vi "GenINI_Main.vi"() -> ()   [LabVIEW 2009]
uses:
  Typedefs/GenINI_Key_Values.ctl
  Typedefs/GenINI_Read_Types.ctl
  Queue/Queue_Type.ctl
  <vilib>/Utility/miscctls.llb/LVPointTypeDef.ctl
panel:
  in  "Exit":bool
  in  "Main Tab":enum32{"Main", "Debug"}(tab)
  in  "Guess types?":bool
  in  "Generate_Typedef":bool
  in  "Generate_Code":bool
  in  "INI file":path=path "C:/"
  in  "Read_INI":bool
  in  "INI read results":T1[](array[typedef])
  in  "error in (no error)":errorcluster
  out "error out":errorcluster
  # "Version: 0.1.0"
  # "1. Select the existing INI file"
  # "2. Set the type for each key, then..."
  # "Name: GenINI\nAuthor: Joe Zoller\nLatest update: Feb. 13th, 2010\nCategory: Scripting\nVersion: 0.1.0\nLabVIEW Version: 2009\nLicense Type: BSD"
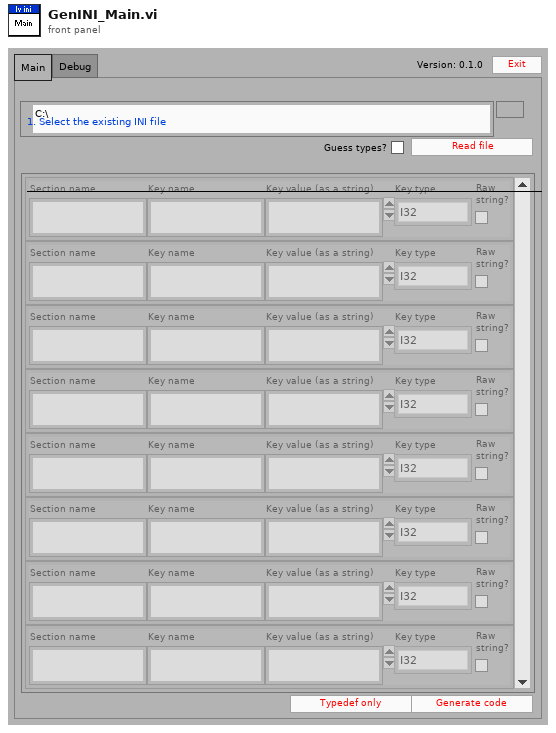
[diagram p1: front panel]
types:
  T1 = typedef "GenINI_Key_Values.ctl" = cluster{"Section name":string, "Key name":string, "Key value (as a string)":string, "Key type":T2, "Raw\nstring?":bool}
  T2 = typedef "GenINI_Read_Types.ctl" = enum16{"Boolean", "Double", "I32", "Path", "String", "U32"}
  T3 = cluster{"typedef path":path, "INI read results":T1[]}
  T4 = typedef "Queue_Type.ctl" = cluster{"cmd":string, "data":variant}
  T5 = typedef "LVPointTypeDef.ctl" = cluster{"Horizontal":i16, "Vertical":i16}
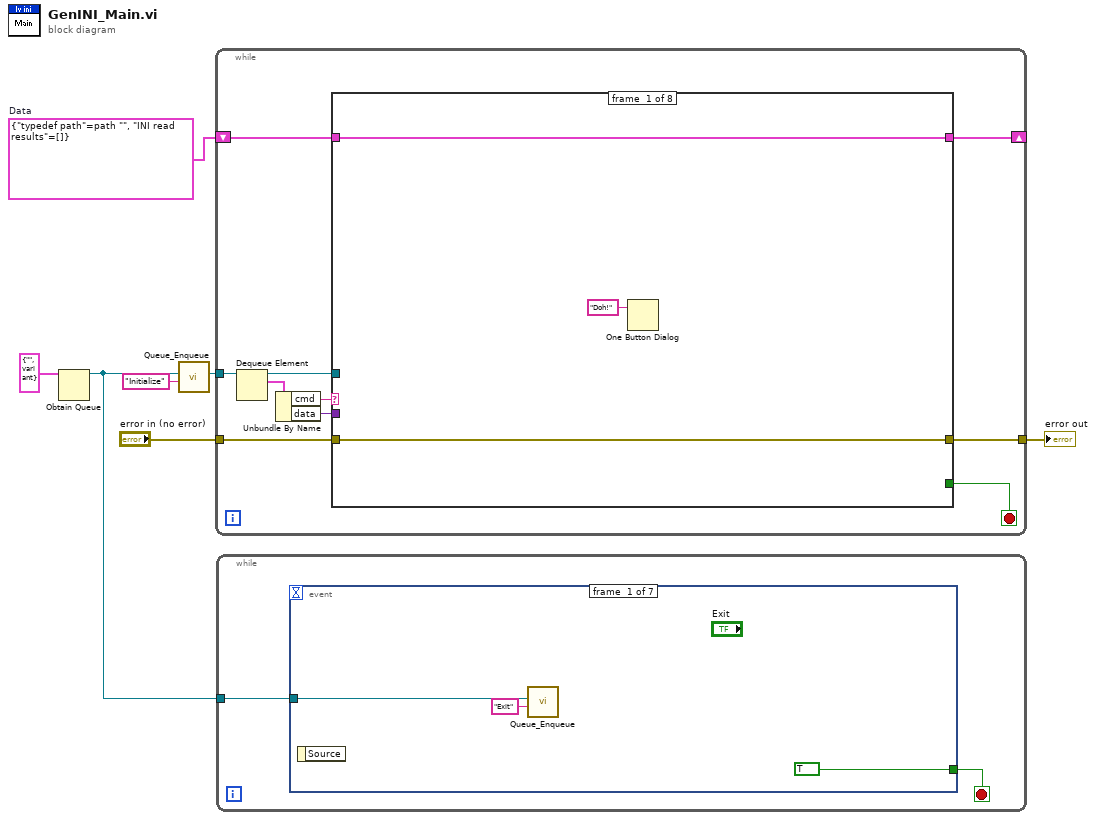
[diagram p0: block diagram]
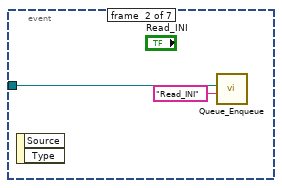
[diagram p2: hidden frame]
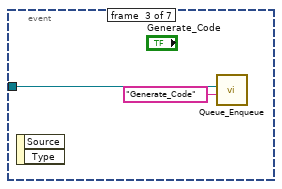
[diagram p3: hidden frame]
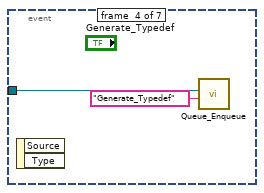
[diagram p4: hidden frame]
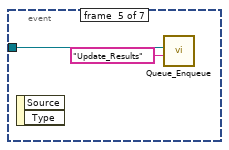
[diagram p5: hidden frame]
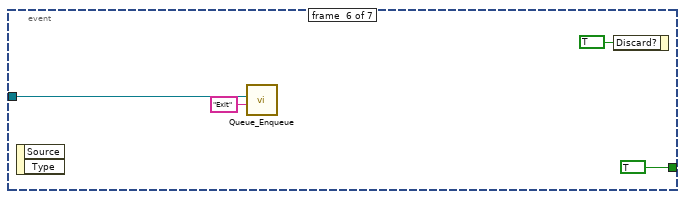
[diagram p6: hidden frame]
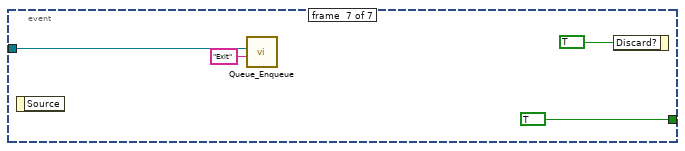
[diagram p7: hidden frame]
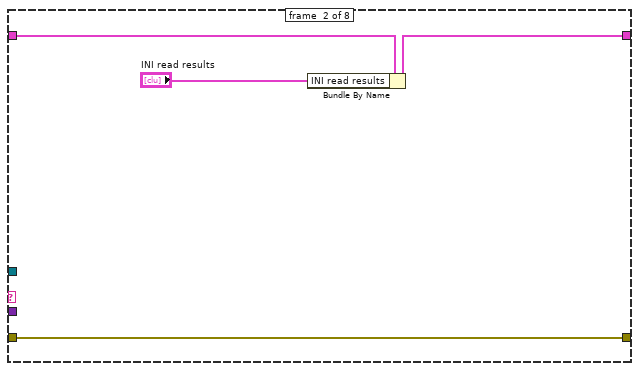
[diagram p8: hidden frame]
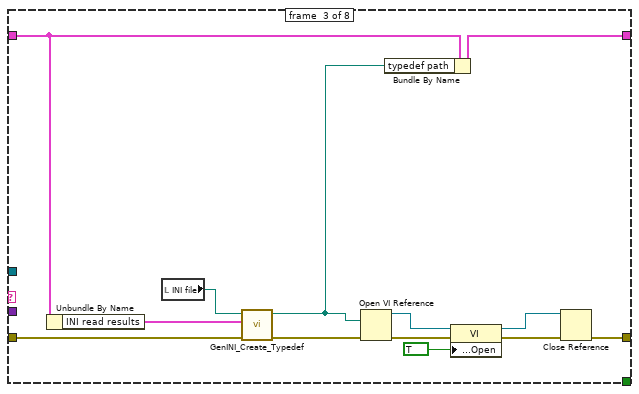
[diagram p9: hidden frame]
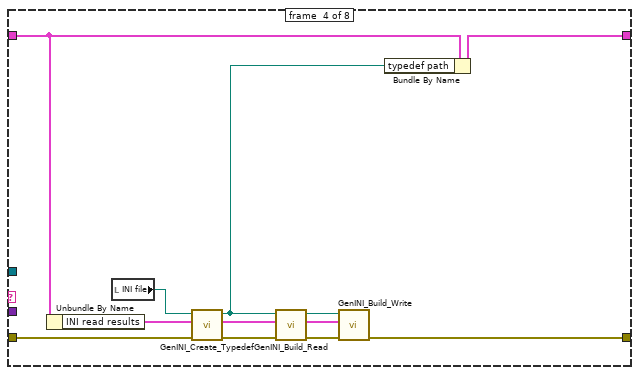
[diagram p10: hidden frame]
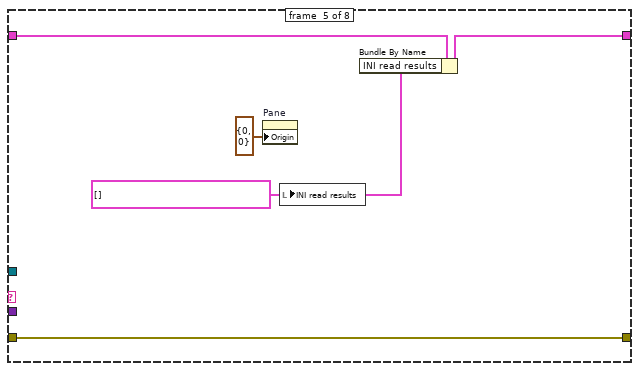
[diagram p11: hidden frame]
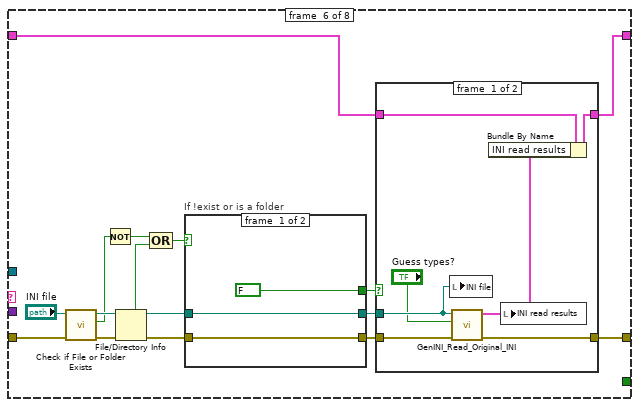
[diagram p12: hidden frame]
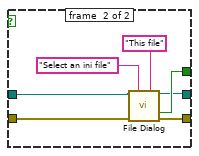
[diagram p13: hidden frame]
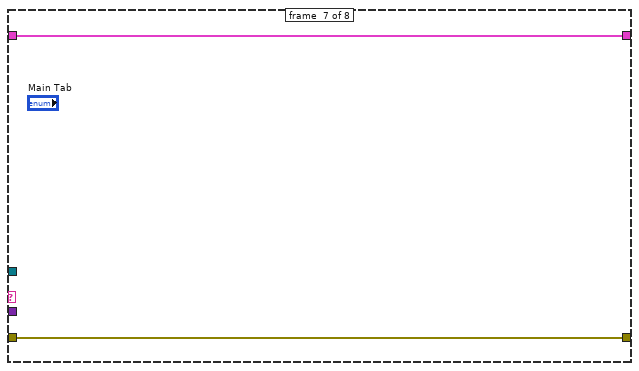
[diagram p15: hidden frame]
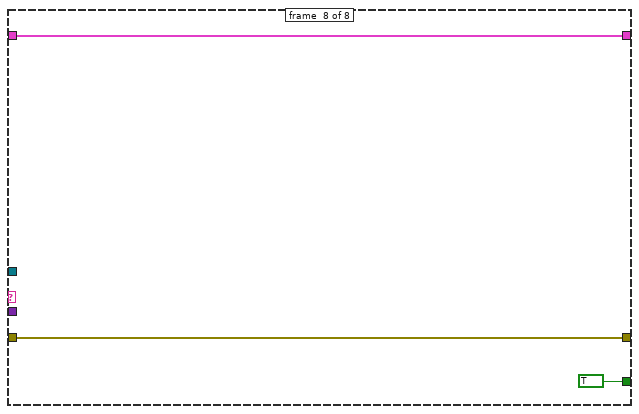
[diagram p16: hidden frame]
diagram:
  w4 = T3 {"typedef path"=path "", "INI read results"=[]}  # Data
  n1 = Obtain Queue(element data type=T4 {"cmd"="", "data"=variant} ("Queue type")) -> (queue out=w3:refnum<queue>)  [unwired: 4 in, 2 out]
  n2 = call "Queue_Enqueue.vi"("cmd"="Initialize", "queue"=w3) -> ("queue out"=w2:refnum<queue>)  [unwired: 8 in, 1 out]
  n3 = while {
    tunnel: w2 -> [w15]
    shift-right: [w10] -> _
    shift-left: w4 -> [w11]
    tunnel: "error in (no error)" -> [w17]
    tunnel: [w16] -> w5
    stop <- w9 stop-if-true
    n4 = Dequeue Element(queue=w15) -> (queue out=w14:refnum<queue>, element=w13:T4)  [unwired: 2 in, 2 out]
    n5 = Unbundle By Name(w13) -> ("cmd"=w12:string, "data"=w8:variant)
    n6 = case shown="\"Initialize\"" w12 {
      tunnel: w17 -> [w20 w24 w36 w48 w54 w67 w91 w94]
      tunnel: [w20 w24 w28 w40 w54 w70 w91 w94] -> w16
      tunnel: w14 -> [_ _ _ _ _ _ _ _]
      tunnel: w11 -> [w18 w23 w26 w46 w52 w56 w90 w93]
      tunnel: [w18 w22 w35 w47 w51 w55 w90 w93] -> w10
      tunnel: [_ _ _ _ _ _ _ TRUE] -> w9
      tunnel: w8 -> [_ _ _ _ _ _ _ _]
      frame #0 {
        n7 = One Button Dialog(message="Doh!") -> ()  [unwired: 1 in, 1 out]
      }
      frame #1 {
        n8 = Bundle By Name(cluster=w23, "INI read results"="INI read results") -> (w22:T3)
      }
      frame #2 {
        n9 = Unbundle By Name(w26) -> ("INI read results"=w25:T1[])
        n10 = local read "INI file"() -> (w37:path)
        n11 = call "GenINI_Create_Typedef.vi"("error in (no error)"=w36, "INI values"=w25, "ini path"=w37) -> ("error out"=w34:errorcluster, "typedef path"=w33:path)  [unwired: 6 in, 1 out]
        n12 = Open VI Reference(vi path=w33, error in (no error)=w34) -> (vi reference=w31:refnum<vi>, error out=w32:errorcluster)  [unwired: 4 in]
        n13 = Bundle By Name(cluster=w26, "typedef path"=w33) -> (w35:T3)
        n14 = property class="VI"(reference=w31, error in=w32, "Front Panel Window:Open"=TRUE) -> (reference out=w27:refnum<vi>, error out=w29:errorcluster)
        n15 = Close Reference(reference=w27, error in (no error)=w29) -> (error out=w28:errorcluster)
      }
      frame #3 {
        n16 = Unbundle By Name(w46) -> ("INI read results"=w43:T1[])
        n17 = local read "INI file"() -> (w49:path)
        n18 = call "GenINI_Create_Typedef.vi"("error in (no error)"=w48, "INI values"=w43, "ini path"=w49) -> ("error out"=w45:errorcluster, "INI values out"=w42:T1[], "typedef path"=w44:path)  [unwired: 6 in]
        n19 = call "GenINI_Build_Read.vi"("error in (no error)"=w45, "INI read values"=w42, "Typedef path"=w44) -> ("error out"=w41:errorcluster, "INI read values dup"=w38:T1[], "Typedef path dup"=w39:path)  [unwired: 6 in]
        n20 = call "GenINI_Build_Write.vi"("error in (no error)"=w41, "INI read values"=w38, "Typedef path"=w39) -> ("error out"=w40:errorcluster)  [unwired: 6 in, 2 out]
        n21 = Bundle By Name(cluster=w46, "typedef path"=w44) -> (w47:T3)
      }
      frame #4 {
        w50 = T1[] [] ("INI read results")
        n22 = property on="Pane" class="Pane"("Origin"=T5 {"Horizontal"=0, "Vertical"=0}) -> ()  [unwired: 2 in, 2 out]
        n23 = local write "INI read results"(w50) -> ()
        n24 = Bundle By Name(cluster=w52, "INI read results"=w50) -> (w51:T3)
      }
      frame #5 {
        n25 = call <vilib>:"Check if File or Folder Exists.vi"("error in (no error)"=w67, "path"="INI file") -> ("error out"=w68:errorcluster, "file or folder exists?"=w65:bool, "dup path"=w66:path)  [unwired: 7 in]
        n26 = Not(x=w65) -> (.not. x?=w64:bool)
        n27 = File/Directory Info(path=w66, error in=w68) -> (path out=w60:path, directory=w63:bool, error out=w62:errorcluster)  [unwired: 4 out]
        n28 = Compound Arithmetic op=OR(w64, w63) -> (w61:bool)
        n29 = case "If !exist or is a folder" shown="True" w61 {
          tunnel: w62 -> [w72 w80]
          tunnel: w60 -> [w73 w78]
          tunnel: [w73 w74] -> w59
          tunnel: [w72 w79] -> w58
          tunnel: [FALSE ("cancelled") w75] -> w57
          frame #0 {
          }
          frame #1 {
            n30 = call "File Dialog"("start path"=w78, "prompt"="Select an ini file", "button label"="This file", "error in"=w80) -> ("selected path"=w74:path, "cancelled"=w75:bool, "error out"=w79:errorcluster)  [unwired: 8 in, 1 out]
          }
        }
        n31 = case shown="False" w57 {
          tunnel: [w87 w89] -> w70
          tunnel: w58 -> [w86 w89]
          tunnel: w59 -> [w85 _]
          tunnel: w56 -> [w84 w88]
          tunnel: [w82 w88] -> w55
          frame #0 {
            n32 = local write "INI file"(w85) -> ()
            n33 = call "GenINI_Read_Original_INI.vi"("error in (no error)"=w86, "Guess types?"="Guess types?", "Path"=w85) -> ("error out"=w87:errorcluster, "Value types"=w83:T1[])  [unwired: 7 in]
            n34 = Bundle By Name(cluster=w84, "INI read results"=w83) -> (w82:T3)
            n35 = local write "INI read results"(w83) -> ()
          }
          frame #1 {
          }
        }
      }
      frame #6 {
      }
      frame #7 {
      }
    }
  }
  "error out" <- w5
  n36 = while {
    tunnel: w3 -> [w96]
    stop <- w95 stop-if-true
    n37 = event shown="[5] Application Instance Close?" {
      selector: _ -> [_ _ _ _ _ _ _]
      dyn-events: _ -> [_ _ _ _ _ _ _]
      timeout: _ -> [_ _ _ _ _ _ _]
      tunnel: w96 -> [w98 w101 w103 w104 w107 w110 w114]
      tunnel: [TRUE _ _ _ _ TRUE TRUE] -> w95
      event #0 {
        n38 = event-data() -> ()  [unwired: 1 in, 1 out]
        n39 = call "Queue_Enqueue.vi"("cmd"="Exit", "queue"=w98) -> ()  [unwired: 8 in, 2 out]
      }
      event #1 {
        n40 = event-data() -> ()  [unwired: 1 in, 2 out]
        n41 = call "Queue_Enqueue.vi"("cmd"="Read_INI", "queue"=w101) -> ()  [unwired: 8 in, 2 out]
      }
      event #2 {
        n42 = event-data() -> ()  [unwired: 1 in, 2 out]
        n43 = call "Queue_Enqueue.vi"("cmd"="Generate_Code", "queue"=w103) -> ()  [unwired: 8 in, 2 out]
      }
      event #3 {
        n44 = event-data() -> ()  [unwired: 1 in, 2 out]
        n45 = call "Queue_Enqueue.vi"("cmd"="Generate_Typedef", "queue"=w104) -> ()  [unwired: 8 in, 2 out]
      }
      event #4 {
        n46 = event-data() -> ()  [unwired: 1 in, 2 out]
        n47 = call "Queue_Enqueue.vi"("cmd"="Update_Results", "queue"=w107) -> ()  [unwired: 8 in, 2 out]
      }
      event #5 {
        n48 = event-data() -> ()  [unwired: 1 in, 2 out]
        n49 = call "Queue_Enqueue.vi"("cmd"="Exit", "queue"=w110) -> ()  [unwired: 8 in, 2 out]
        n50 = event-data("Discard?"=TRUE) -> ()  [unwired: 1 in, 1 out]
      }
      event #6 {
        n51 = event-data() -> ()  [unwired: 1 in, 1 out]
        n52 = call "Queue_Enqueue.vi"("cmd"="Exit", "queue"=w114) -> ()  [unwired: 8 in, 2 out]
        n53 = event-data("Discard?"=TRUE) -> ()  [unwired: 1 in, 1 out]
      }
    }
  }
